vi "PQmakeEmptyPGresult.vi"(0 "conn":u64, 1 "status":i64, 3 "error in (no error)":errorcluster) -> (7 "conn_out":u64, 8 "res":u64, 10 "error out":errorcluster)   [LabVIEW 2019, in "libpqlv64.lvlib"]
doc: "Constructs an empty PGresult object with the given status."
uses:
  libpqlv64.lvlib
  libpq.dll
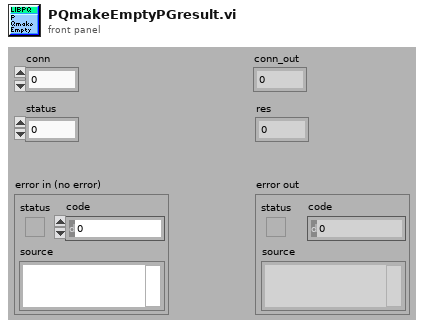
[diagram p1: front panel]
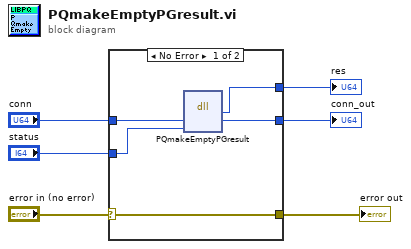
[diagram p0: block diagram]
diagram:
  n1 = case shown="No Error" "error in (no error)" {
    selector: "error in (no error)" -> [w11 w13]
    tunnel: [w11 w13] -> w5
    tunnel: [w10 _] -> w4
    tunnel: "status" -> [w9 _]
    tunnel: "conn" -> [w8 w12]
    tunnel: [w7 w12] -> w1
    frame No Error {
      n2 = dll-call lib="libpq.*" fn="PQmakeEmptyPGresult"("conn"=w8, "status"=w9) -> ("res"=w10:u64, "conn"=w7:u64)  [unwired: 4 in, 2 out]
    }
    frame Error {
    }
  }
  "res" <- w4
  "error out" <- w5
  "conn_out" <- w1
